vi "Teste3.vi"() -> ()   [LabVIEW 2012]
uses:
  Application/Application.lvclass
  RxTXCamera/RxTxCamera.lvclass
  CCDCamera.lvclass
  Application/Application.lvclass/Application.ctl
  RxTx/RxTx.lvclass/RxTx.ctl
  Instrument/Instrument.lvclass/Instrument.ctl
  State Machine/State Machine.lvclass/State Machine.ctl
  CCDCamera.lvclass/CCDCamera.ctl
  RxTXCamera/RxTxCamera.lvclass/RxTxCamera.ctl
  Construct String Header/Construct String Header.lvclass/Construct String Header.ctl
  RxTx/Write Message.vi
  RxTXCamera/Write Construct String Header.lvclass.vi
  RxTXCamera/Read Construct String Header.lvclass.vi
  Construct String Header/Write Header Contents.vi
  Construct String Header/Make string.vi
  State Machine/State Machine.lvclass
  Construct String Header/Construct String Header.lvclass
  Instrument/Instrument.lvclass
  RxTx/RxTx.lvclass
panel:
  in  "CCDCamera in":refnum<class "CCDCamera.lvclass">
  in  "RxTxCamera.lvclass":refnum<class "RxTxCamera.lvclass">
  in  "Application in":refnum<class "Application.lvclass">
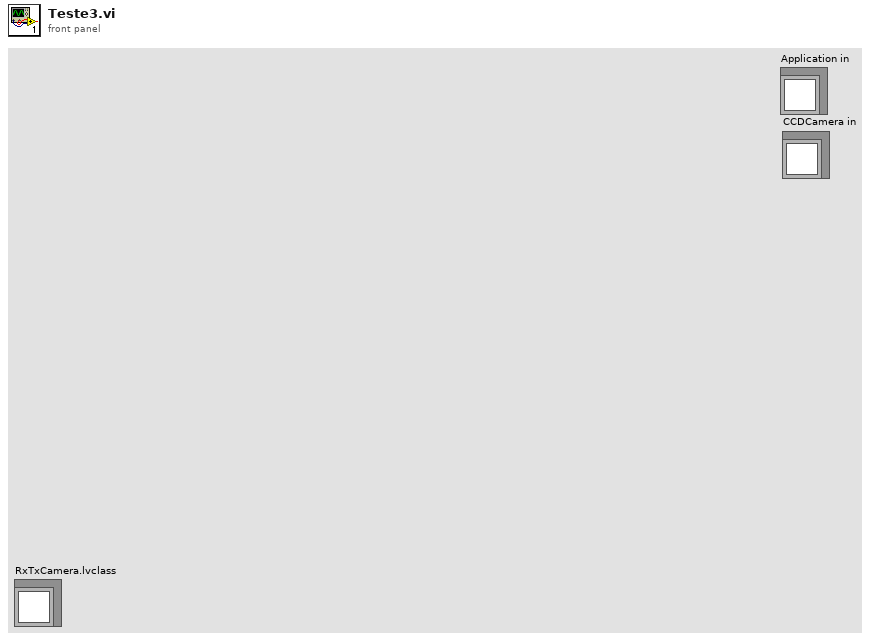
[diagram p1: front panel]
types:
  T1 = cluster{"Currently Temperature":dbl, "Last Image":string, "% Acquired":dbl, "Initilizarion":bool, "Exposing":bool, "Temperature Status":string, "X length":dbl, "Y length":dbl, "Min Temperature":dbl, "Max Temperature":dbl}
  T2 = cluster{"FILENAME":string[], "OBSERVER":string[], "PROGRID":string[], "OBJECT":string[], "NIGHTDIR":string[], "CHANNEL":string[], "INSTRUME":string[], "NEXPSEQ":string[], "SEQINDEX":string[], "OBSTYPE":string[], "READMOD":string[], "SHUTTER":string[], "OPENSHT":string[], "CLOSESHT":string[], "GAIN":string[], "GAINERR ":string[], "RDNOISE":string[], "RNOISERR":string[], "SKYFIBER":string[], "CALFIBER":string[], "UTDATE":string[], "LOCTIME":string[], "MJD":string[], "OBSLON":string[], "OBSLAT":string[], "OBSALT":string[], "EXPTIME":string[], "TELRA":string[], "TELDEC":string[], "RA":string[], "DEC":string[], "RA_DEG":string[], "DEC_DEG":string[], "EPOCH":string[], "HA":string[], "HAD":string[], "AIRMASS":string[], "AMSTART":string[], "AMEND":string[], "XOFFSET":string[], "YOFFSET":string[], "PA":string[], "CAMFOC":string[], "TELFOC":string[], "TCSUT":string[], "MOONDIST":string[], "MOONALT":string[], "MONNPHAS":string[], "ADC":string[], "ADCSPPED":string[], "CALMIRR":string[], "GUIDING":string[], "GUIDTEXP":string[], "GUIDFREQ":string[], "GUIDOBJX":string[], "GUIDOBJY":string[], "AVGYCORR":string[], "AVGXCORR":string[], "GFOCUS":string[], "THARLAMP":string[], "HALLAMP":string[], "AGITATOR":string[], "THARMIRR":string[], "DSTATUS":string[], "DTEMP":string[], "DHUM":string[], "DLAMP":string[], "DFLAT":string[], "TEMPEXT":string[], "PRESSURE":string[], "HUMIDITY":string[], "WINDDIR":string[], "WSPEED":string[], "TCSST":string[], "DPOS":string[]}
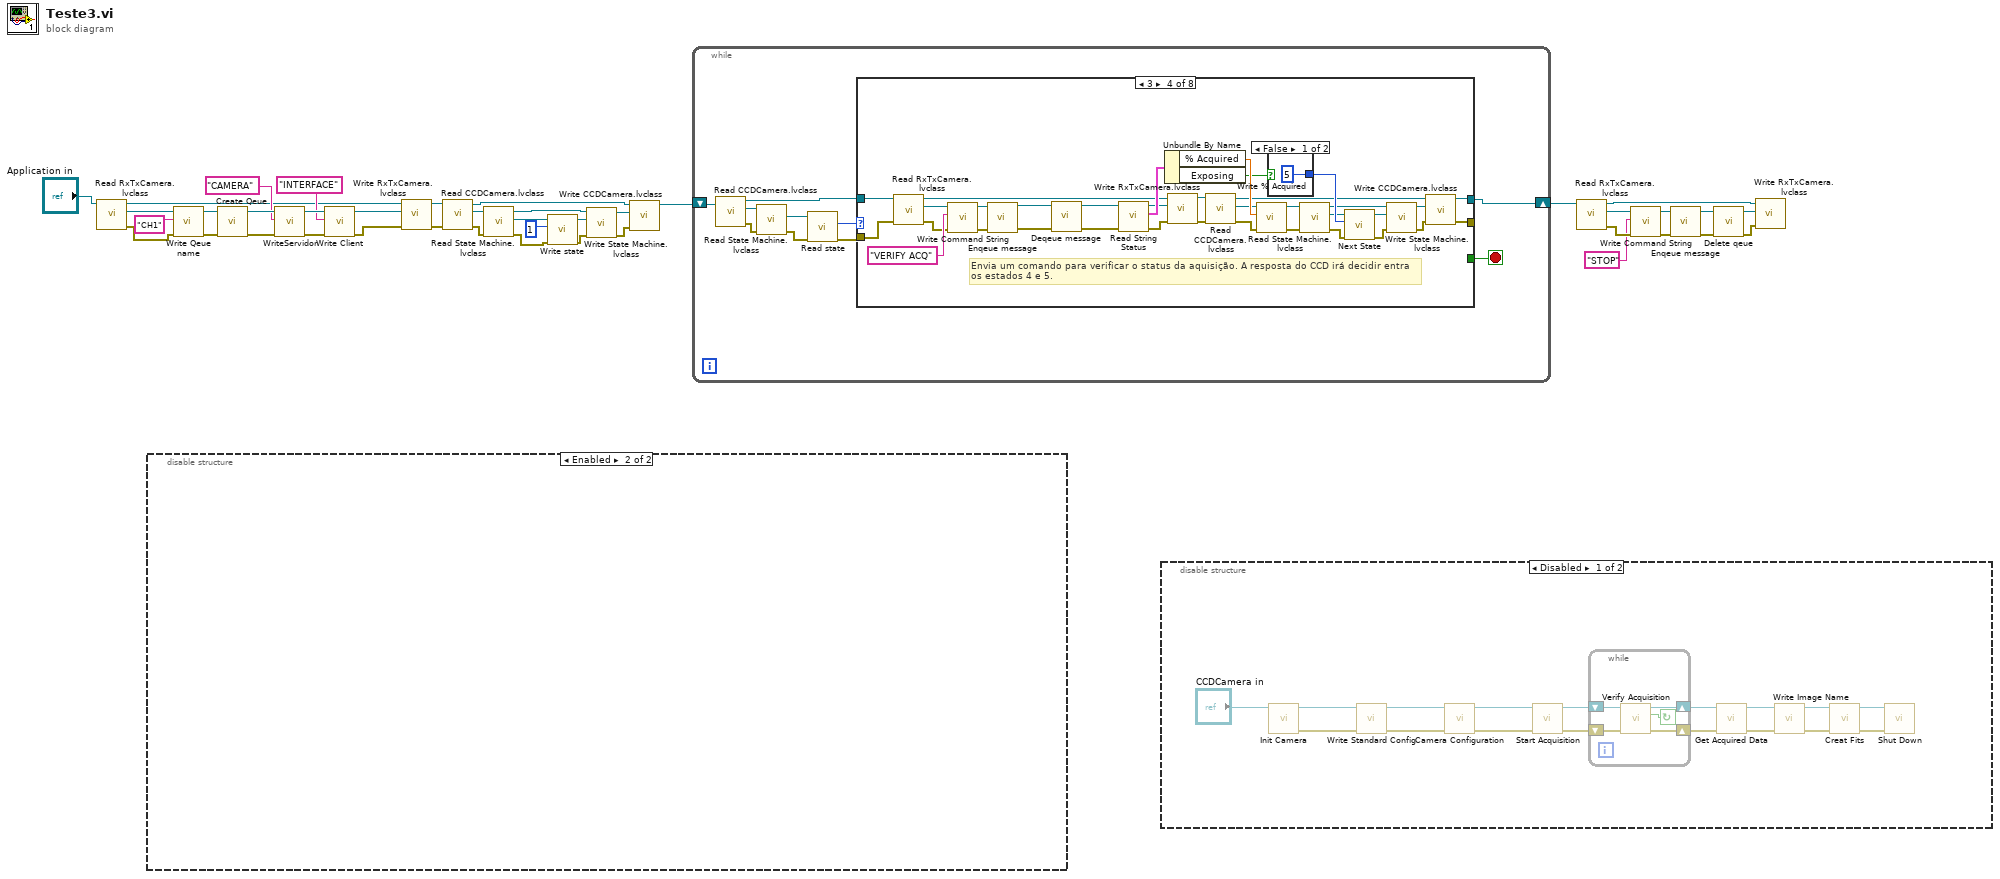
[diagram p0: block diagram]
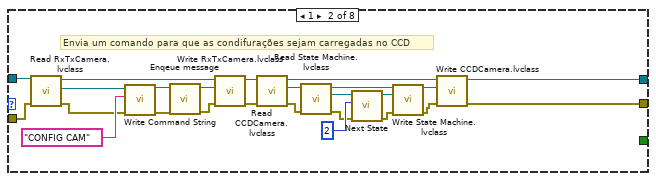
[diagram p3: hidden frame]
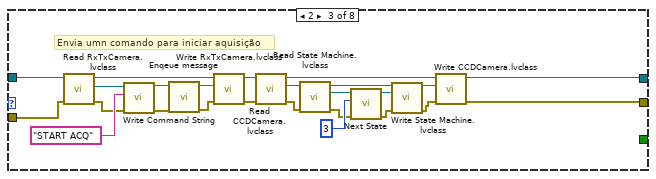
[diagram p4: hidden frame]
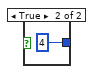
[diagram p5: hidden frame]
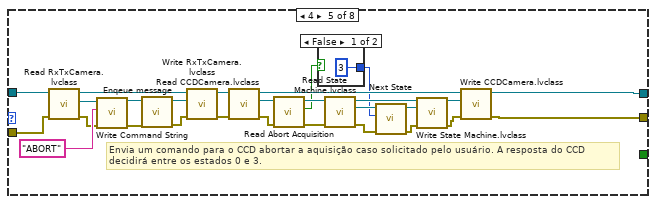
[diagram p6: hidden frame]
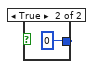
[diagram p7: hidden frame]
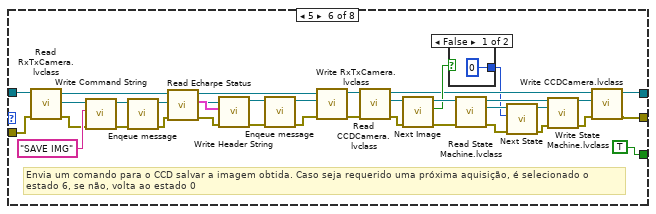
[diagram p8: hidden frame]
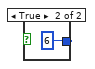
[diagram p9: hidden frame]
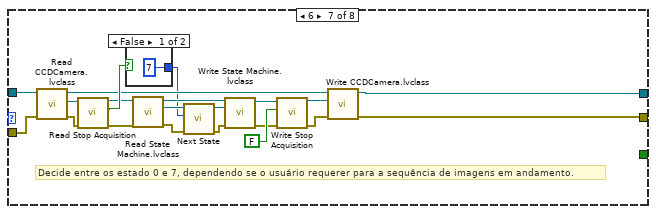
[diagram p10: hidden frame]
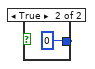
[diagram p11: hidden frame]
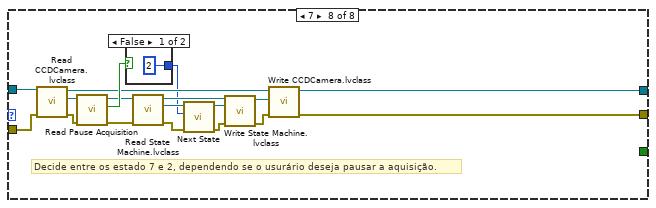
[diagram p12: hidden frame]
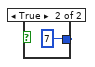
[diagram p13: hidden frame]
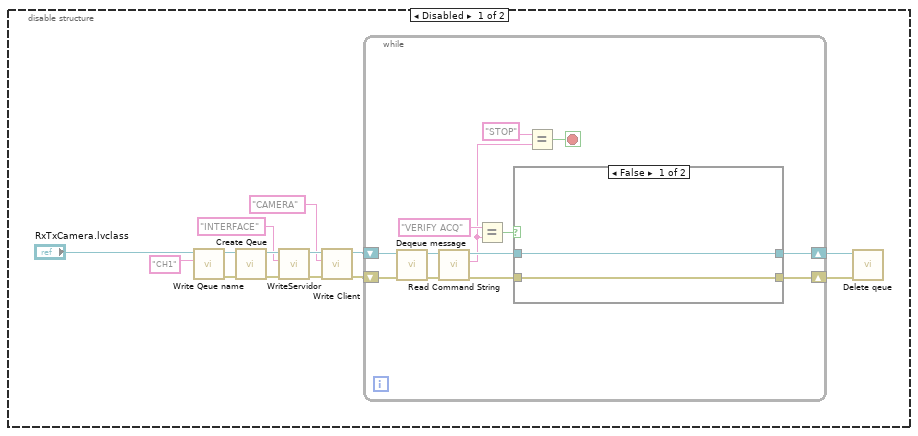
[diagram p15: hidden frame]
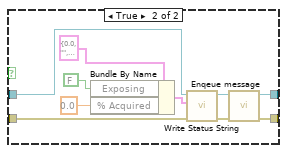
[diagram p16: hidden frame]
diagram:
  n1 = call "Read RxTxCamera.lvclass.vi"("Application in"="Application in") -> ("error out"=w26:errorcluster, "RxTxCamera.lvclass"=w31:refnum<class "RxTxCamera.lvclass">, "Application out"=w28:refnum<class "Application.lvclass">)  [unwired: 8 in]
  n2 = disable-structure shown="Enabled" {
    frame Disabled {
      n3 = call "Write Qeue name.vi"("Qeue name"="CH1", "RxTx in"="RxTxCamera.lvclass") -> ("error out"=w52:errorcluster, "RxTx out"=w53:refnum<class "RxTxCamera.lvclass">)  [unwired: 8 in]
      n4 = call "Create Qeue.vi"("error in (no error)"=w52, "RxTx in"=w53) -> ("error out"=w47:errorcluster, "RxTx out"=w48:refnum<class "RxTxCamera.lvclass">)  [unwired: 8 in]
      n5 = call "WriteServidor.vi"("error in (no error)"=w47, "Servidor"="INTERFACE" ("Qeue name"), "RxTx in"=w48) -> ("error out"=w50:errorcluster, "RxTx out"=w49:refnum<class "RxTxCamera.lvclass">)  [unwired: 7 in]
      n6 = call "Write Client.vi"("error in (no error)"=w50, "Client"="CAMERA" ("Qeue name"), "RxTx in"=w49) -> ("error out"=w43:errorcluster, "RxTx out"=w44:refnum<class "RxTxCamera.lvclass">)  [unwired: 7 in]
      n7 = while {
        shift-right: [w58] -> w41
        shift-left: w44 -> [w67]
        shift-right: [w59] -> w42
        shift-left: w43 -> [w66]
        stop <- w56 stop-if-true
        n8 = call "Deqeue message.vi"("error in (no error)"=w66, "RxTx in"=w67) -> ("error out"=w65:errorcluster, "RxTx out"=w64:refnum<class "RxTxCamera.lvclass">)  [unwired: 8 in]
        n9 = call "Read Command String.vi"("error in (no error)"=w65, "RxTxCamera in"=w64) -> ("error out"=w60:errorcluster, "String Command"=w55:string, "RxTxCamera out"=w61:refnum<class "RxTxCamera.lvclass">)  [unwired: 7 in]
        n10 = Equal?(x="VERIFY ACQ", y=w55) -> (x = y?=w63:bool)
        n11 = case shown="False" w63 {
          tunnel: w61 -> [w69 w73]
          tunnel: w60 -> [w68 w72]
          tunnel: [w68 w71] -> w59
          tunnel: [w69 w70] -> w58
          frame False {
          }
          frame True {
            n12 = Bundle By Name(cluster=T1 {"Currently Temperature"=0.0, "Last Image"="", "% Acquired"=0.0, "Initilizarion"=FALSE, "Exposing"=FALSE, "Temperature Status"="", "X length"=0.0, "Y length"=0.0, "Min Temperature"=0.0, "Max Temperature"=0.0} ("Camera Status"), "Exposing"=FALSE, "% Acquired"=0.0) -> (w78:T1)
            n13 = call "Write Status String.vi"("error in (no error)"=w72, "Camera Status"=w78, "RxTxCamera in"=w73) -> ("error out"=w76:errorcluster, "RxTxCamera out"=w77:refnum<class "RxTxCamera.lvclass">)  [unwired: 7 in]
            n14 = call "Enqeue message.vi"("error in (no error)"=w76, "RxTx in"=w77) -> ("error out"=w71:errorcluster, "RxTx out"=w70:refnum<class "RxTxCamera.lvclass">)  [unwired: 8 in]
          }
        }
        n15 = Equal?(x="STOP", y=w55) -> (x = y?=w56:bool)
      }
      n16 = call "Delete qeue.vi"("error in (no error)"=w42, "RxTx in"=w41) -> ()  [unwired: 8 in, 2 out]
    }
    frame Enabled {
    }
  }
  n17 = call "Write Qeue name.vi"("error in (no error)"=w26, "Qeue name"="CH1", "RxTx in"=w31) -> ("error out"=w38:errorcluster, "RxTx out"=w39:refnum<class "RxTxCamera.lvclass">)  [unwired: 7 in]
  n18 = call "Create Qeue.vi"("error in (no error)"=w38, "RxTx in"=w39) -> ("error out"=w34:errorcluster, "RxTx out"=w35:refnum<class "RxTxCamera.lvclass">)  [unwired: 8 in]
  n19 = call "WriteServidor.vi"("error in (no error)"=w34, "Servidor"="CAMERA" ("Qeue name"), "RxTx in"=w35) -> ("error out"=w37:errorcluster, "RxTx out"=w36:refnum<class "RxTxCamera.lvclass">)  [unwired: 7 in]
  n20 = call "Write Client.vi"("error in (no error)"=w37, "Client"="INTERFACE" ("Qeue name"), "RxTx in"=w36) -> ("error out"=w27:errorcluster, "RxTx out"=w29:refnum<class "RxTxCamera.lvclass">)  [unwired: 7 in]
  n21 = call "Write RxTxCamera.lvclass.vi"("error in (no error)"=w27, "RxTxCamera.lvclass"=w29, "Application in"=w28) -> ("error out"=w20:errorcluster, "Application out"=w19:refnum<class "Application.lvclass">)  [unwired: 7 in]
  n22 = call "Read CCDCamera.lvclass.vi"("error in (no error)"=w20, "Application in"=w19) -> ("error out"=w22:errorcluster, "CCDCamera.lvclass"=w21:refnum<class "CCDCamera.lvclass">, "Application out"=w13:refnum<class "Application.lvclass">)  [unwired: 7 in]
  n23 = call "Read State Machine.lvclass.vi"("error in (no error)"=w22, "Instrument in"=w21) -> ("error out"=w24:errorcluster, "State Machine.lvclass"=w23:refnum<class "State Machine.lvclass">, "Instrument out"=w16:refnum<class "CCDCamera.lvclass">)  [unwired: 7 in]
  n24 = call "Write state.vi"("error in (no error)"=w24, "state"=u32 1, "State Machine in"=w23) -> ("error out"=w18:errorcluster, "State Machine out"=w17:refnum<class "State Machine.lvclass">)  [unwired: 7 in]
  n25 = call "Write State Machine.lvclass.vi"("error in (no error)"=w18, "State Machine.lvclass"=w17, "Instrument in"=w16) -> ("error out"=w15:errorcluster, "Instrument out"=w14:refnum<class "CCDCamera.lvclass">)  [unwired: 7 in]
  n26 = call "Write CCDCamera.lvclass.vi"("error in (no error)"=w15, "CCDCamera.lvclass"=w14, "Application in"=w13) -> ("Application out"=w12:refnum<class "Application.lvclass">)  [unwired: 7 in, 1 out]
  n27 = while {
    shift-right: [w81] -> w6
    shift-left: w12 -> [w87]
    stop <- w80 stop-if-true
    n28 = call "Read CCDCamera.lvclass.vi"("Application in"=w87) -> ("error out"=w88:errorcluster, "CCDCamera.lvclass"=w89:refnum<class "CCDCamera.lvclass">, "Application out"=w84:refnum<class "Application.lvclass">)  [unwired: 8 in]
    n29 = call "Read State Machine.lvclass.vi"("error in (no error)"=w88, "Instrument in"=w89) -> ("error out"=w86:errorcluster, "State Machine.lvclass"=w85:refnum<class "State Machine.lvclass">)  [unwired: 7 in, 1 out]
    n30 = call "Read state.vi"("error in (no error)"=w86, "State Machine in"=w85) -> ("error out"=w82:errorcluster, "state"=w83:u32)  [unwired: 7 in, 1 out]
    n31 = case shown="3" w83 {
      tunnel: w82 -> [w90 w116 w119 w174 w186 w215 w248 w271]
      tunnel: w84 -> [w91 w115 w120 w175 w187 w216 w249 w272]
      tunnel: [w91 w93 w118 w143 w179 w229 w246 w270] -> w81
      tunnel: [w90 w92 w117 w142 w178 w228 w247 w269] -> _
      tunnel: [_ _ _ _ _ TRUE _ _] -> w80
      frame 0, Default {
      }
      frame 1 {
        # "Envia um comando para que as condifurações sejam carregadas no CCD"
        n32 = call "Read RxTxCamera.lvclass.vi"("error in (no error)"=w116, "Application in"=w115) -> ("error out"=w107:errorcluster, "RxTxCamera.lvclass"=w109:refnum<class "RxTxCamera.lvclass">, "Application out"=w113:refnum<class "Application.lvclass">)  [unwired: 7 in]
        n33 = call "Write Command String.vi"("error in (no error)"=w107, "Command String"="CONFIG CAM", "RxTxCamera in"=w109) -> ("error out"=w112:errorcluster, "RxTxCamera out"=w111:refnum<class "RxTxCamera.lvclass">)  [unwired: 7 in]
        n34 = call "Enqeue message.vi"("error in (no error)"=w112, "RxTx in"=w111) -> ("error out"=w114:errorcluster, "RxTx out"=w110:refnum<class "RxTxCamera.lvclass">)  [unwired: 8 in]
        n35 = call "Write RxTxCamera.lvclass.vi"("error in (no error)"=w114, "RxTxCamera.lvclass"=w110, "Application in"=w113) -> ("error out"=w106:errorcluster, "Application out"=w105:refnum<class "Application.lvclass">)  [unwired: 7 in]
        n36 = call "Read CCDCamera.lvclass.vi"("error in (no error)"=w106, "Application in"=w105) -> ("error out"=w104:errorcluster, "CCDCamera.lvclass"=w103:refnum<class "CCDCamera.lvclass">, "Application out"=w96:refnum<class "Application.lvclass">)  [unwired: 7 in]
        n37 = call "Read State Machine.lvclass.vi"("error in (no error)"=w104, "Instrument in"=w103) -> ("error out"=w101:errorcluster, "State Machine.lvclass"=w100:refnum<class "State Machine.lvclass">, "Instrument out"=w97:refnum<class "CCDCamera.lvclass">)  [unwired: 7 in]
        n38 = call "Next State.vi"("error in (no error)"=w101, "New_State"=u32 2, "State Machine in"=w100) -> ("error out"=w99:errorcluster, "State Machine out"=w98:refnum<class "State Machine.lvclass">)  [unwired: 7 in]
        n39 = call "Write State Machine.lvclass.vi"("error in (no error)"=w99, "State Machine.lvclass"=w98, "Instrument in"=w97) -> ("error out"=w95:errorcluster, "Instrument out"=w94:refnum<class "CCDCamera.lvclass">)  [unwired: 7 in]
        n40 = call "Write CCDCamera.lvclass.vi"("error in (no error)"=w95, "CCDCamera.lvclass"=w94, "Application in"=w96) -> ("error out"=w92:errorcluster, "Application out"=w93:refnum<class "Application.lvclass">)  [unwired: 7 in]
      }
      frame 2 {
        # "Envia umn comando para iniciar aquisição"
        n41 = call "Read RxTxCamera.lvclass.vi"("error in (no error)"=w119, "Application in"=w120) -> ("error out"=w134:errorcluster, "RxTxCamera.lvclass"=w136:refnum<class "RxTxCamera.lvclass">, "Application out"=w140:refnum<class "Application.lvclass">)  [unwired: 7 in]
        n42 = call "Write Command String.vi"("error in (no error)"=w134, "Command String"="START ACQ", "RxTxCamera in"=w136) -> ("error out"=w139:errorcluster, "RxTxCamera out"=w138:refnum<class "RxTxCamera.lvclass">)  [unwired: 7 in]
        n43 = call "Enqeue message.vi"("error in (no error)"=w139, "RxTx in"=w138) -> ("error out"=w141:errorcluster, "RxTx out"=w137:refnum<class "RxTxCamera.lvclass">)  [unwired: 8 in]
        n44 = call "Write RxTxCamera.lvclass.vi"("error in (no error)"=w141, "RxTxCamera.lvclass"=w137, "Application in"=w140) -> ("error out"=w133:errorcluster, "Application out"=w132:refnum<class "Application.lvclass">)  [unwired: 7 in]
        n45 = call "Read CCDCamera.lvclass.vi"("error in (no error)"=w133, "Application in"=w132) -> ("error out"=w131:errorcluster, "CCDCamera.lvclass"=w130:refnum<class "CCDCamera.lvclass">, "Application out"=w123:refnum<class "Application.lvclass">)  [unwired: 7 in]
        n46 = call "Read State Machine.lvclass.vi"("error in (no error)"=w131, "Instrument in"=w130) -> ("error out"=w128:errorcluster, "State Machine.lvclass"=w127:refnum<class "State Machine.lvclass">, "Instrument out"=w124:refnum<class "CCDCamera.lvclass">)  [unwired: 7 in]
        n47 = call "Next State.vi"("error in (no error)"=w128, "New_State"=u32 3, "State Machine in"=w127) -> ("error out"=w126:errorcluster, "State Machine out"=w125:refnum<class "State Machine.lvclass">)  [unwired: 7 in]
        n48 = call "Write State Machine.lvclass.vi"("error in (no error)"=w126, "State Machine.lvclass"=w125, "Instrument in"=w124) -> ("error out"=w122:errorcluster, "Instrument out"=w121:refnum<class "CCDCamera.lvclass">)  [unwired: 7 in]
        n49 = call "Write CCDCamera.lvclass.vi"("error in (no error)"=w122, "CCDCamera.lvclass"=w121, "Application in"=w123) -> ("error out"=w117:errorcluster, "Application out"=w118:refnum<class "Application.lvclass">)  [unwired: 7 in]
      }
      frame 3 {
        # "Envia um comando para verificar o status da aquisição. A resposta do CCD irá decidir entra\nos estados 4 e 5."
        n50 = call "Read RxTxCamera.lvclass.vi"("error in (no error)"=w174, "Application in"=w175) -> ("error out"=w167:errorcluster, "RxTxCamera.lvclass"=w168:refnum<class "RxTxCamera.lvclass">, "Application out"=w161:refnum<class "Application.lvclass">)  [unwired: 7 in]
        n51 = call "Write Command String.vi"("error in (no error)"=w167, "Command String"="VERIFY ACQ", "RxTxCamera in"=w168) -> ("error out"=w170:errorcluster, "RxTxCamera out"=w166:refnum<class "RxTxCamera.lvclass">)  [unwired: 7 in]
        n52 = call "Enqeue message.vi"("error in (no error)"=w170, "RxTx in"=w166) -> ("error out"=w165:errorcluster, "RxTx out"=w164:refnum<class "RxTxCamera.lvclass">)  [unwired: 8 in]
        n53 = call "Deqeue message.vi"("error in (no error)"=w165, "RxTx in"=w164) -> ("error out"=w173:errorcluster, "RxTx out"=w172:refnum<class "RxTxCamera.lvclass">)  [unwired: 8 in]
        n54 = call "Read String Status.vi"("error in (no error)"=w173, "RxTxCamera in"=w172) -> ("error out"=w163:errorcluster, "Camera Status"=w171:T1, "RxTxCamera out"=w162:refnum<class "RxTxCamera.lvclass">)  [unwired: 7 in]
        n55 = Unbundle By Name(w171) -> ("% Acquired"=w158:dbl, "Exposing"=w151:bool)
        n56 = call "Write RxTxCamera.lvclass.vi"("error in (no error)"=w163, "RxTxCamera.lvclass"=w162, "Application in"=w161) -> ("error out"=w160:errorcluster, "Application out"=w159:refnum<class "Application.lvclass">)  [unwired: 7 in]
        n57 = call "Read CCDCamera.lvclass.vi"("error in (no error)"=w160, "Application in"=w159) -> ("error out"=w156:errorcluster, "CCDCamera.lvclass"=w157:refnum<class "CCDCamera.lvclass">, "Application out"=w144:refnum<class "Application.lvclass">)  [unwired: 7 in]
        n58 = call "Write % Acquired.vi"("error in (no error)"=w156, "% Acquired"=w158, "CCDCamera in"=w157) -> ("error out"=w153:errorcluster, "CCDCamera out"=w152:refnum<class "CCDCamera.lvclass">)  [unwired: 7 in]
        n59 = case shown="False" w151 {
          tunnel: [u32 5 ("New_State") u32 4 ("New_State")] -> w150
          frame False {
          }
          frame True {
          }
        }
        n60 = call "Read State Machine.lvclass.vi"("error in (no error)"=w153, "Instrument in"=w152) -> ("error out"=w155:errorcluster, "State Machine.lvclass"=w149:refnum<class "State Machine.lvclass">, "Instrument out"=w147:refnum<class "CCDCamera.lvclass">)  [unwired: 7 in]
        n61 = call "Next State.vi"("error in (no error)"=w155, "New_State"=w150, "State Machine in"=w149) -> ("error out"=w154:errorcluster, "State Machine out"=w148:refnum<class "State Machine.lvclass">)  [unwired: 7 in]
        n62 = call "Write State Machine.lvclass.vi"("error in (no error)"=w154, "State Machine.lvclass"=w148, "Instrument in"=w147) -> ("error out"=w146:errorcluster, "Instrument out"=w145:refnum<class "CCDCamera.lvclass">)  [unwired: 7 in]
        n63 = call "Write CCDCamera.lvclass.vi"("error in (no error)"=w146, "CCDCamera.lvclass"=w145, "Application in"=w144) -> ("error out"=w142:errorcluster, "Application out"=w143:refnum<class "Application.lvclass">)  [unwired: 7 in]
      }
      frame 4 {
        # "Envia um comando para o CCD abortar a aquisição caso solicitado pelo usuário. A resposta do CCD\ndecidirá entre os estados 0 e 3."
        n64 = call "Read RxTxCamera.lvclass.vi"("error in (no error)"=w186, "Application in"=w187) -> ("error out"=w198:errorcluster, "RxTxCamera.lvclass"=w200:refnum<class "RxTxCamera.lvclass">, "Application out"=w204:refnum<class "Application.lvclass">)  [unwired: 7 in]
        n65 = call "Write Command String.vi"("error in (no error)"=w198, "Command String"="ABORT", "RxTxCamera in"=w200) -> ("error out"=w203:errorcluster, "RxTxCamera out"=w202:refnum<class "RxTxCamera.lvclass">)  [unwired: 7 in]
        n66 = call "Enqeue message.vi"("error in (no error)"=w203, "RxTx in"=w202) -> ("error out"=w205:errorcluster, "RxTx out"=w201:refnum<class "RxTxCamera.lvclass">)  [unwired: 8 in]
        n67 = call "Write RxTxCamera.lvclass.vi"("error in (no error)"=w205, "RxTxCamera.lvclass"=w201, "Application in"=w204) -> ("error out"=w197:errorcluster, "Application out"=w196:refnum<class "Application.lvclass">)  [unwired: 7 in]
        n68 = call "Read CCDCamera.lvclass.vi"("error in (no error)"=w197, "Application in"=w196) -> ("error out"=w184:errorcluster, "CCDCamera.lvclass"=w185:refnum<class "CCDCamera.lvclass">, "Application out"=w190:refnum<class "Application.lvclass">)  [unwired: 7 in]
        n69 = call "Read Abort Acquisition.vi"("error in (no error)"=w184, "CCDCamera in"=w185) -> ("error out"=w183:errorcluster, "Abort Acquisition"=w181:bool, "CCDCamera out"=w182:refnum<class "CCDCamera.lvclass">)  [unwired: 7 in]
        n70 = case shown="False" w181 {
          tunnel: [u32 3 ("New_State") u32 0 ("New_State")] -> w180
          frame False {
          }
          frame True {
          }
        }
        n71 = call "Read State Machine.lvclass.vi"("error in (no error)"=w183, "Instrument in"=w182) -> ("error out"=w195:errorcluster, "State Machine.lvclass"=w194:refnum<class "State Machine.lvclass">, "Instrument out"=w191:refnum<class "CCDCamera.lvclass">)  [unwired: 7 in]
        n72 = call "Next State.vi"("error in (no error)"=w195, "New_State"=w180, "State Machine in"=w194) -> ("error out"=w193:errorcluster, "State Machine out"=w192:refnum<class "State Machine.lvclass">)  [unwired: 7 in]
        n73 = call "Write State Machine.lvclass.vi"("error in (no error)"=w193, "State Machine.lvclass"=w192, "Instrument in"=w191) -> ("error out"=w189:errorcluster, "Instrument out"=w188:refnum<class "CCDCamera.lvclass">)  [unwired: 7 in]
        n74 = call "Write CCDCamera.lvclass.vi"("error in (no error)"=w189, "CCDCamera.lvclass"=w188, "Application in"=w190) -> ("error out"=w178:errorcluster, "Application out"=w179:refnum<class "Application.lvclass">)  [unwired: 7 in]
      }
      frame 5 {
        # "Envia um comando para o CCD salvar a imagem obtida. Caso seja requerido uma próxima aquisição, é selecionado o \nestado 6, se não, volta ao estado 0"
        n75 = call "Read RxTxCamera.lvclass.vi"("error in (no error)"=w215, "Application in"=w216) -> ("error out"=w213:errorcluster, "RxTxCamera.lvclass"=w212:refnum<class "RxTxCamera.lvclass">, "Application out"=w220:refnum<class "Application.lvclass">)  [unwired: 7 in]
        n76 = call "Write Command String.vi"("error in (no error)"=w213, "Command String"="SAVE IMG", "RxTxCamera in"=w212) -> ("error out"=w211:errorcluster, "RxTxCamera out"=w209:refnum<class "RxTxCamera.lvclass">)  [unwired: 7 in]
        n77 = call "Enqeue message.vi"("error in (no error)"=w211, "RxTx in"=w209) -> ("error out"=w210:errorcluster, "RxTx out"=w208:refnum<class "RxTxCamera.lvclass">)  [unwired: 8 in]
        n78 = call "Read Echarpe Status.vi"("error in (no error)"=w210, "Application in"=w220) -> ("error out"=w223:errorcluster, "Header Contents out"=w222:T2, "Application out"=w221:refnum<class "Application.lvclass">)  [unwired: 7 in]
        n79 = call "Write Header String.vi"("error in (no error)"=w223, "Header Contents"=w222, "RxTxCamera in"=w208) -> ("error out"=w224:errorcluster, "RxTxCamera out"=w225:refnum<class "RxTxCamera.lvclass">)  [unwired: 7 in]
        n80 = call "Enqeue message.vi"("error in (no error)"=w224, "RxTx in"=w225) -> ("error out"=w226:errorcluster, "RxTx out"=w227:refnum<class "RxTxCamera.lvclass">)  [unwired: 8 in]
        n81 = call "Write RxTxCamera.lvclass.vi"("error in (no error)"=w226, "RxTxCamera.lvclass"=w227, "Application in"=w221) -> ("error out"=w218:errorcluster, "Application out"=w217:refnum<class "Application.lvclass">)  [unwired: 7 in]
        n82 = call "Read CCDCamera.lvclass.vi"("error in (no error)"=w218, "Application in"=w217) -> ("error out"=w239:errorcluster, "CCDCamera.lvclass"=w240:refnum<class "CCDCamera.lvclass">, "Application out"=w233:refnum<class "Application.lvclass">)  [unwired: 7 in]
        n83 = call "Next Image"("error in (no error)"=w239, "CCDCamera in"=w240) -> ("error out"=w243:errorcluster, "Next Image ?"=w241:bool, "CCDCamera out"=w242:refnum<class "CCDCamera.lvclass">)  [unwired: 7 in]
        n84 = case shown="False" w241 {
          tunnel: [u32 0 ("New_State") u32 6 ("New_State")] -> w230
          frame False {
          }
          frame True {
          }
        }
        n85 = call "Read State Machine.lvclass.vi"("error in (no error)"=w243, "Instrument in"=w242) -> ("error out"=w238:errorcluster, "State Machine.lvclass"=w237:refnum<class "State Machine.lvclass">, "Instrument out"=w234:refnum<class "CCDCamera.lvclass">)  [unwired: 7 in]
        n86 = call "Next State.vi"("error in (no error)"=w238, "New_State"=w230, "State Machine in"=w237) -> ("error out"=w236:errorcluster, "State Machine out"=w235:refnum<class "State Machine.lvclass">)  [unwired: 7 in]
        n87 = call "Write State Machine.lvclass.vi"("error in (no error)"=w236, "State Machine.lvclass"=w235, "Instrument in"=w234) -> ("error out"=w232:errorcluster, "Instrument out"=w231:refnum<class "CCDCamera.lvclass">)  [unwired: 7 in]
        n88 = call "Write CCDCamera.lvclass.vi"("error in (no error)"=w232, "CCDCamera.lvclass"=w231, "Application in"=w233) -> ("error out"=w228:errorcluster, "Application out"=w229:refnum<class "Application.lvclass">)  [unwired: 7 in]
      }
      frame 6 {
        # "Decide entre os estado 0 e 7, dependendo se o usuário requerer para a sequência de imagens em andamento."
        n89 = call "Read CCDCamera.lvclass.vi"("error in (no error)"=w248, "Application in"=w249) -> ("error out"=w258:errorcluster, "CCDCamera.lvclass"=w257:refnum<class "CCDCamera.lvclass">, "Application out"=w251:refnum<class "Application.lvclass">)  [unwired: 7 in]
        n90 = call "Read Stop Acquisition.vi"("error in (no error)"=w258, "CCDCamera in"=w257) -> ("error out"=w259:errorcluster, "Stop Acquisition"=w261:bool, "CCDCamera out"=w260:refnum<class "CCDCamera.lvclass">)  [unwired: 7 in]
        n91 = case shown="False" w261 {
          tunnel: [u32 7 ("New_State") u32 0 ("New_State")] -> w250
          frame False {
          }
          frame True {
          }
        }
        n92 = call "Read State Machine.lvclass.vi"("error in (no error)"=w259, "Instrument in"=w260) -> ("error out"=w256:errorcluster, "State Machine.lvclass"=w255:refnum<class "State Machine.lvclass">, "Instrument out"=w252:refnum<class "CCDCamera.lvclass">)  [unwired: 7 in]
        n93 = call "Next State.vi"("error in (no error)"=w256, "New_State"=w250, "State Machine in"=w255) -> ("error out"=w254:errorcluster, "State Machine out"=w253:refnum<class "State Machine.lvclass">)  [unwired: 7 in]
        n94 = call "Write State Machine.lvclass.vi"("error in (no error)"=w254, "State Machine.lvclass"=w253, "Instrument in"=w252) -> ("error out"=w262:errorcluster, "Instrument out"=w263:refnum<class "CCDCamera.lvclass">)  [unwired: 7 in]
        n95 = call "Write Stop Acquisition.vi"("error in (no error)"=w262, "Stop Acquisition"=FALSE, "CCDCamera in"=w263) -> ("error out"=w264:errorcluster, "CCDCamera out"=w265:refnum<class "CCDCamera.lvclass">)  [unwired: 7 in]
        n96 = call "Write CCDCamera.lvclass.vi"("error in (no error)"=w264, "CCDCamera.lvclass"=w265, "Application in"=w251) -> ("error out"=w247:errorcluster, "Application out"=w246:refnum<class "Application.lvclass">)  [unwired: 7 in]
      }
      frame 7 {
        # "Decide entre os estado 7 e 2, dependendo se o usurário deseja pausar a aquisição."
        n97 = call "Read CCDCamera.lvclass.vi"("error in (no error)"=w271, "Application in"=w272) -> ("error out"=w280:errorcluster, "CCDCamera.lvclass"=w281:refnum<class "CCDCamera.lvclass">, "Application out"=w274:refnum<class "Application.lvclass">)  [unwired: 7 in]
        n98 = call "Read Pause Acquisition.vi"("error in (no error)"=w280, "CCDCamera in"=w281) -> ("error out"=w282:errorcluster, "Pause Acquisition"=w284:bool, "CCDCamera out"=w283:refnum<class "CCDCamera.lvclass">)  [unwired: 7 in]
        n99 = case shown="False" w284 {
          tunnel: [u32 2 ("New_State") u32 7 ("New_State")] -> w273
          frame False {
          }
          frame True {
          }
        }
        n100 = call "Read State Machine.lvclass.vi"("error in (no error)"=w282, "Instrument in"=w283) -> ("error out"=w279:errorcluster, "State Machine.lvclass"=w278:refnum<class "State Machine.lvclass">, "Instrument out"=w275:refnum<class "CCDCamera.lvclass">)  [unwired: 7 in]
        n101 = call "Next State.vi"("error in (no error)"=w279, "New_State"=w273, "State Machine in"=w278) -> ("error out"=w277:errorcluster, "State Machine out"=w276:refnum<class "State Machine.lvclass">)  [unwired: 7 in]
        n102 = call "Write State Machine.lvclass.vi"("error in (no error)"=w277, "State Machine.lvclass"=w276, "Instrument in"=w275) -> ("error out"=w285:errorcluster, "Instrument out"=w286:refnum<class "CCDCamera.lvclass">)  [unwired: 7 in]
        n103 = call "Write CCDCamera.lvclass.vi"("error in (no error)"=w285, "CCDCamera.lvclass"=w286, "Application in"=w274) -> ("error out"=w269:errorcluster, "Application out"=w270:refnum<class "Application.lvclass">)  [unwired: 7 in]
      }
    }
  }
  n104 = disable-structure shown="Disabled" {
    frame Disabled {
      n105 = call "Init Camera.vi"("CCDCamera in"="CCDCamera in") -> ("error out"=w305:errorcluster, "CCDCamera out"=w294:refnum<class "CCDCamera.lvclass">)  [unwired: 9 in]
      n106 = call "Write Standard Config.vi"("error in (no error)"=w305, "CCDCamera in"=w294) -> ("error out"=w304:errorcluster, "CCDCamera out"=w295:refnum<class "CCDCamera.lvclass">)  [unwired: 8 in]
      n107 = call "Camera Configuration.vi"("error in (no error)"=w304, "CCDCamera in"=w295) -> ("error out"=w303:errorcluster, "CCDCamera out"=w296:refnum<class "CCDCamera.lvclass">)  [unwired: 8 in]
      n108 = call "Start Acquisition.vi"("error in (no error)"=w303, "CCDCamera in"=w296) -> ("error out"=w302:errorcluster, "CCDCamera out"=w297:refnum<class "CCDCamera.lvclass">)  [unwired: 8 in]
      n109 = while {
        shift-right: [w308] -> w289
        shift-left: w297 -> [w307]
        shift-right: [w309] -> w292
        shift-left: w302 -> [w310]
        stop <- w306 continue-if-true
        n110 = call "Verify Acquisition.vi"("error in (no error)"=w310, "CCDCamera in"=w307) -> ("error out"=w309:errorcluster, "Acquiring"=w306:bool, "CCDCamera out"=w308:refnum<class "CCDCamera.lvclass">)  [unwired: 7 in]
      }
      n111 = call "Get Acquired Data.vi"("error in (no error)"=w292, "CCDCamera in"=w289) -> ("error out"=w291:errorcluster, "CCDCamera out"=w290:refnum<class "CCDCamera.lvclass">)  [unwired: 8 in]
      n112 = call "Write Image Name.vi"("error in (no error)"=w291, "CCDCamera in"=w290) -> ("error out"=w301:errorcluster, "CCDCamera out"=w298:refnum<class "CCDCamera.lvclass">)  [unwired: 8 in]
      n113 = call "Creat Fits.vi"("error in (no error)"=w301, "CCDCamera in"=w298) -> ("error out"=w300:errorcluster, "CCDCamera out"=w299:refnum<class "CCDCamera.lvclass">)  [unwired: 8 in]
      n114 = call "Shut Down.vi"("error in (no error)"=w300, "CCDCamera in"=w299) -> ()  [unwired: 8 in, 2 out]
    }
    frame Enabled {
    }
  }
  n115 = call "Read RxTxCamera.lvclass.vi"("Application in"=w6) -> ("error out"=w10:errorcluster, "RxTxCamera.lvclass"=w9:refnum<class "RxTxCamera.lvclass">, "Application out"=w1:refnum<class "Application.lvclass">)  [unwired: 8 in]
  n116 = call "Write Command String.vi"("error in (no error)"=w10, "Command String"="STOP", "RxTxCamera in"=w9) -> ("error out"=w7:errorcluster, "RxTxCamera out"=w11:refnum<class "RxTxCamera.lvclass">)  [unwired: 7 in]
  n117 = call "Enqeue message.vi"("error in (no error)"=w7, "RxTx in"=w11) -> ("error out"=w5:errorcluster, "RxTx out"=w4:refnum<class "RxTxCamera.lvclass">)  [unwired: 8 in]
  n118 = call "Delete qeue.vi"("error in (no error)"=w5, "RxTx in"=w4) -> ("error out"=w3:errorcluster, "RxTx out"=w2:refnum<class "RxTxCamera.lvclass">)  [unwired: 8 in]
  n119 = call "Write RxTxCamera.lvclass.vi"("error in (no error)"=w3, "RxTxCamera.lvclass"=w2, "Application in"=w1) -> ()  [unwired: 7 in, 2 out]
